vi "Port Selection.vi"(9 "Coupler Selection":T2, 10 "Incident Selection":T1, 11 "FPT_SParam_Switching in":refnum<class "FPT_SParam_Switching.lvclass">) -> (2 "Coupler Port":string, 3 "Incident Port":string)   [LabVIEW 2023, in "FPT_SParam_Switching.lvclass"]
uses:
  FPT_SParam_Switching.lvclass
  FPT_SParam_Switching.lvclass/FPT_SParam_Switching.ctl
  <vilib>/niSPML/Switching/2 Couplers Per Port 1 VST/Coupler Selection.ctl
  <vilib>/niSPML/Switching/2 Couplers Per Port 1 VST/S-Par 2 Couplers Per Port 1 VST Switching.lvclass
  <vilib>/niSPML/Switching/2 Couplers Per Port 1 VST/Incident Selection.ctl
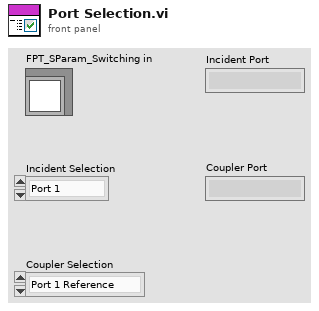
[diagram p1: front panel]
types:
  T1 = typedef "S-Par Switching.lvlib/S-Par 2 Couplers Per Port 1 VST Switching.lvclass/Incident Selection.ctl" = enum16{"Port 1", "Port 2"}
  T2 = typedef "S-Par Switching.lvlib/S-Par 2 Couplers Per Port 1 VST Switching.lvclass/Coupler Selection.ctl" = enum16{"Port 1 Reference", "Port 1 Test", "Port 2 Reference", "Port 2 Test"}
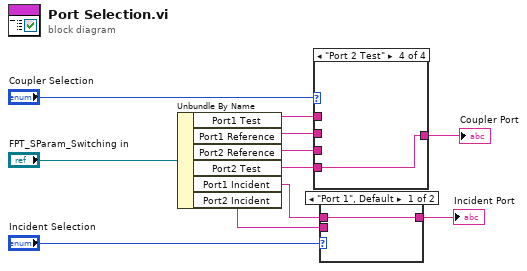
[diagram p0: block diagram]
diagram:
  n1 = Unbundle By Name("FPT_SParam_Switching in") -> ("Port1 Test"=w9:string, "Port1 Reference"=w8:string, "Port2 Reference"=w7:string, "Port2 Test"=w6:string, "Port1 Incident"=w4:string, "Port2 Incident"=w3:string)
  n2 = case shown="\"Port 2 Test\"" "Coupler Selection" {
    tunnel: [w12 w13 w14 w15] -> w11
    tunnel: w9 -> [_ w13 _ _]
    tunnel: w8 -> [w12 _ _ _]
    tunnel: w7 -> [_ _ w14 _]
    tunnel: w6 -> [_ _ _ w15]
    frame "Port 1 Reference", Default {
    }
    frame "Port 1 Test" {
    }
    frame "Port 2 Reference" {
    }
    frame "Port 2 Test" {
    }
  }
  "Coupler Port" <- w11
  n3 = case shown="\"Port 1\", Default" "Incident Selection" {
    tunnel: w4 -> [w16 _]
    tunnel: w3 -> [_ w17]
    tunnel: [w16 w17] -> w2
    frame "Port 1", Default {
    }
    frame "Port 2" {
    }
  }
  "Incident Port" <- w2
